vi "DataType Cacher(DT).vi"(7 "GroupName(\"\")":string, 9 "Type":T1, 10 "key":string) -> (0 "error out":errorcluster, 2 "stored type":T1, 3 "match?":bool, 6 "cacher":variant)   [LabVIEW 2017]
uses:
  <vilib>/Utility/Data Type/Type Definitions/Data Type.ctl
  9d131c6f-10be-47fc-9827-901a6724fd55.vi
  <vilib>/Utility/Data Type/NI_Data Type.lvlib
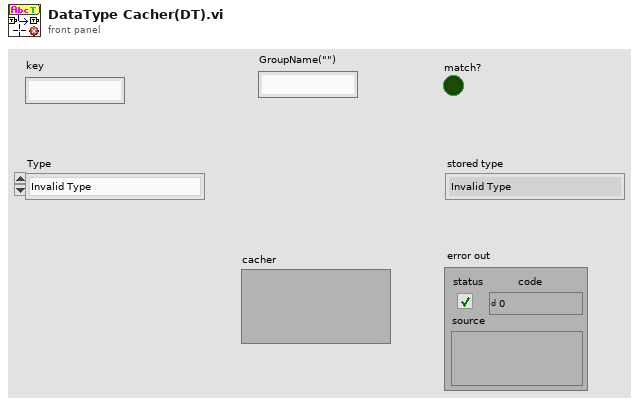
[diagram p1: front panel]
types:
  T1 = typedef "NI_Data Type.lvlib/Data Type.ctl" = enum8{"Invalid Type", "Void", "I8", "I16", "I32", "I64", "U8", "U16", "U32", "U64", "Single Float", "Double Float", "Extended Float", "Single Complex", "Double Complex", "Extended Complex", "Enum U8", "Enum U16", "Enum U32", "Enum U64", "Single Float With Unit", "Double Float With Unit", "Extended Float With Unit", "Single Complex with Unit", "Double Complex with Unit", "Extended Complex with Unit", "Boolean", "String", "Path", "Picture", "Tag", "Array", "Cluster", "Variant", "LV Variant", "Waveform", "Timestamp", "Digital Waveform", "Digital Data", "ExpressData", "Refnum", "External Data", "VI", "Poly VI", "LabVIEW Class Instance", "Fixed Point"}
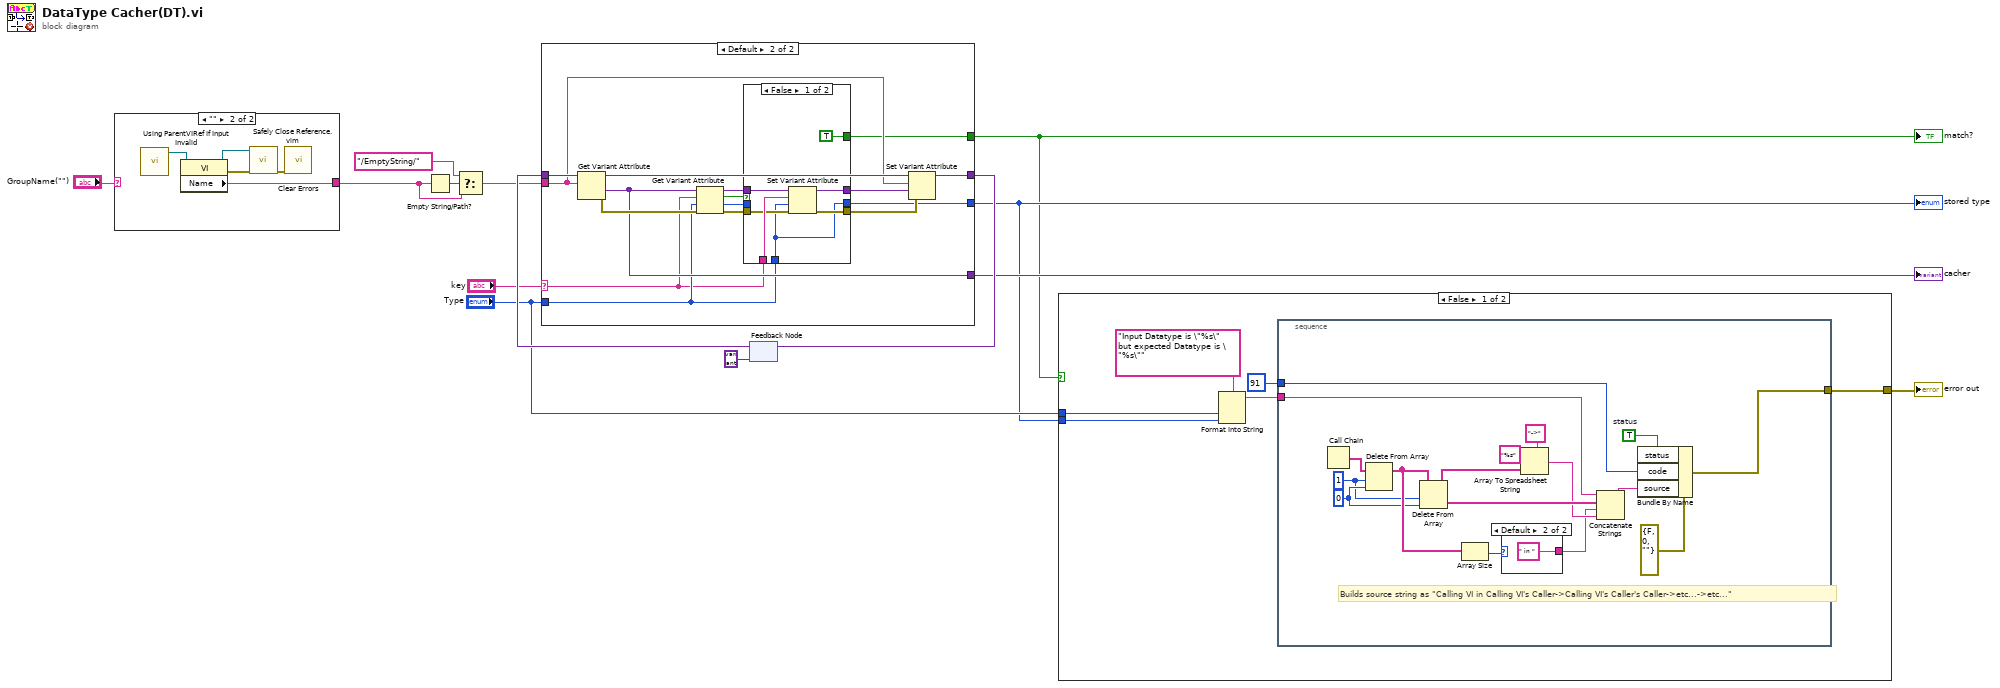
[diagram p0: block diagram]
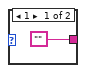
[diagram p3: hidden frame]
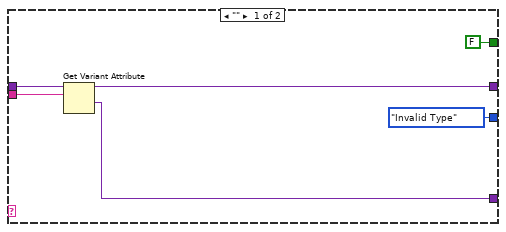
[diagram p5: hidden frame]
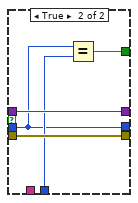
[diagram p6: hidden frame]
diagram:
  n1 = case shown="\"\"" "GroupName(\"\")" {
    selector: "GroupName(\"\")" -> [w15 _]
    tunnel: [w15 w17] -> w1
    frame "False", Default {
    }
    frame "" {
      n2 = call "Using ParentVIRef If Input Invalid.vi"() -> ("VI Ref"=w16:refnum<vi>)  [unwired: 6 in, 1 out]
      n3 = property class="VI"(reference=w16) -> (reference out=w19:refnum<vi>, error out=w18:errorcluster, "Name"=w17:string)  [unwired: 1 in]
      n4 = call "Safely Close Reference.vim"("error in (no error)"=w18, "Reference"=w19) -> ("error out"=w20:errorcluster)  [unwired: 9 in]
      n5 = call <vilib>:"Clear Errors.vi"("error in (no error)"=w20) -> ()  [unwired: 5 in, 2 out]
    }
  }
  n6 = Empty String/Path?(string/path=w1) -> (empty?=w13:bool)
  n7 = Select(t="/EmptyString/", s=w13, f=w1) -> (s? t:f=w10:string)
  n8 = feedback #1(variant) -> (w11:variant)
  n9 = case shown="Default" "key" {
    selector: "key" -> [_ w29]
    tunnel: w11 -> [w25 w38]
    tunnel: w10 -> [w26 w35]
    tunnel: [w24 w32] -> w9
    tunnel: [w23 w31] -> w8
    tunnel: "Type" -> [_ w30]
    tunnel: [FALSE w28] -> w3
    tunnel: [Data_Type."Invalid Type" ("Type") w27] -> w4
    frame "" {
      n10 = Get Variant Attribute(Variant=w25, name=w26) -> (duplicate Variant=w24:variant, value=w23:variant)  [unwired: 2 in, 2 out]
    }
    frame Default {
      n11 = Get Variant Attribute(Variant=w38, name=w35) -> (duplicate Variant=w37:variant, value=w31:variant, error out=w34:errorcluster)  [unwired: 2 in, 1 out]
      n12 = Get Variant Attribute(Variant=w31, name=w29, default value (empty Variant)=w30, error in=w34) -> (duplicate Variant=w42:variant, found=w41:bool, value=w40:T1, error out=w39:errorcluster)
      n13 = case shown="False" w41 {
        tunnel: w42 -> [w49 w54]
        tunnel: w29 -> [w48 _]
        tunnel: w40 -> [_ w50]
        tunnel: w39 -> [w47 w53]
        tunnel: [w46 w54] -> w36
        tunnel: [w45 w53] -> w33
        tunnel: w30 -> [w43 w52]
        tunnel: [TRUE w51] -> w28
        tunnel: [w43 w50] -> w27
        frame False {
          n14 = Set Variant Attribute(Variant=w49, name=w48, value=w43, error in=w47) -> (Variant out=w46:variant, error out=w45:errorcluster)  [unwired: 1 out]
        }
        frame True {
          n15 = Equal?(x=w50, y=w52) -> (x = y?=w51:bool)
        }
      }
      n16 = Set Variant Attribute(Variant=w37, name=w35, value=w36, error in=w33) -> (Variant out=w32:variant)  [unwired: 2 out]
    }
  }
  "cacher" <- w8
  "match?" <- w3
  "stored type" <- w4
  n17 = feedback-in #1(w9) -> ()
  n18 = case shown="False" w3 {
    tunnel: [w60 _] -> w6
    tunnel: "Type" -> [w56 _]
    tunnel: w4 -> [w55 _]
    frame False {
      n19 = Format Into String(format string="Input Datatype is \"%s\" but expected Datatype is \"%s\"", w56, w55) -> (resulting string=w57:string)  [unwired: 2 in, 1 out]
      n20 = stacked-sequence {
        tunnel: [w73] -> w60
        tunnel: w57 -> [w74]
        tunnel: 91 ("code") -> [w70]
        frame #0 {
          w67 = 0 ("Index")
          w66 = 1 ("Length")
          w71 = TRUE  # status
          # "Builds source string as \"Calling VI in Calling VI's Caller->Calling VI's Caller's Caller->etc...->etc...\""
          n21 = Call Chain() -> (call chain=w61:string[])
          n22 = Delete From Array(array=w61, length=w66, index=w67) -> (array with subset deleted=w77:string[])  [unwired: 1 out]
          n23 = Delete From Array(array=w77, length=w66, index=w67) -> (deleted portion=w76:string[], array with subset deleted=w68:string[])
          n24 = Array Size(array=w77) -> (size(s)=w75:i32)
          n25 = case shown="Default" w75 {
            tunnel: ["" " in " ("Format String")] -> w63
            frame 1 {
            }
            frame Default {
            }
          }
          n26 = Array To Spreadsheet String(delimiter (Tab)="->", array=w68, 3:"%s" ("format string")) -> (spreadsheet string=w64:string)
          n27 = Concatenate Strings(w74, w76, w63, w64) -> (w72:string)
          n28 = Bundle By Name(cluster=errorcluster {"status"=FALSE, "code"=0, "source"=""} ("error out"), "status"=w71, "code"=w70, "source"=w72) -> (w73:errorcluster)
        }
      }
    }
    frame True {
    }
  }
  "error out" <- w6
